vi "magnet ami connect.vi"(8 "error in (no error)":errorcluster, 10 "Z-Axis Communications Config":T1={"GPIB address"=22, "GPIB bus"=0, "connection ID"=refnum, "IP"="111.111.111.1", "Active Comm Interface"=0, "Serial Port"="", "Programmer Type"=0} {"Programmer Type" items=["Model 430", "Model 420"]; "Active Comm Interface" items=["TCP/IP (Model 430 Only)", "RS232", "IEEE488"]}, 11 "Y-Axis Communications Config":T1={"GPIB address"=22, "GPIB bus"=0, "connection ID"=refnum, "IP"="111.111.111.2", "Active Comm Interface"=0, "Serial Port"="", "Programmer Type"=0} {"Programmer Type" items=["Model 430", "Model 420"]; "Active Comm Interface" items=["TCP/IP (Model 430 Only)", "RS232", "IEEE488"]}) -> (0 "error out":errorcluster, 2 "Z-Axis Communications Config Out":T1={"GPIB address"=22, "GPIB bus"=0, "connection ID"=refnum, "IP"="111.111.111.1", "Active Comm Interface"=0, "Serial Port"="", "Programmer Type"=0} {"Programmer Type" items=["Model 430", "Model 420"]; "Active Comm Interface" items=["TCP/IP (Model 430 Only)", "RS232", "IEEE488"]}, 3 "Y-Axis Communications Config Out":T1={"GPIB address"=22, "GPIB bus"=0, "connection ID"=refnum, "IP"="111.111.111.2", "Active Comm Interface"=0, "Serial Port"="", "Programmer Type"=0} {"Programmer Type" items=["Model 430", "Model 420"]; "Active Comm Interface" items=["TCP/IP (Model 430 Only)", "RS232", "IEEE488"]})   [LabVIEW 2018]
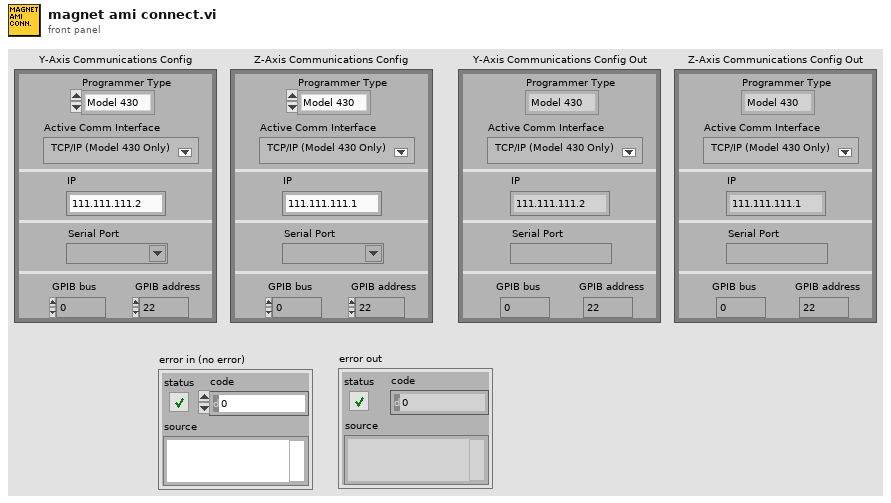
[diagram p1: front panel]
types:
  T1 = cluster{"GPIB address":i16, "GPIB bus":i16, "connection ID":refnum<k5>, "IP":string, "Active Comm Interface":u16, "Serial Port":refnum<visa-resource-name>, "Programmer Type":u16}
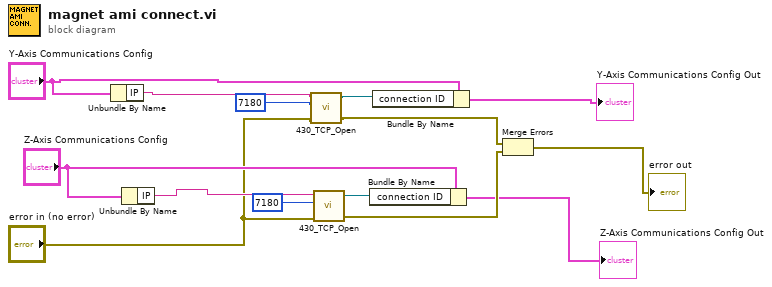
[diagram p0: block diagram]
diagram:
  n1 = Unbundle By Name("Y-Axis Communications Config") -> ("IP"=w8:string)
  n2 = Unbundle By Name("Z-Axis Communications Config") -> ("IP"=w6:string)
  n3 = call "430_TCP_Open.vi"("IP Address"=w8, "TCP Port"=7180, "error in (no error)"="error in (no error)") -> ("connection ID"=w10:refnum<k5>, "error out"=w9:errorcluster)  [unwired: 3 in, 1 out]
  n4 = call "430_TCP_Open.vi"("IP Address"=w6, "TCP Port"=7180, "error in (no error)"="error in (no error)") -> ("connection ID"=w13:refnum<k5>, "error out"=w12:errorcluster)  [unwired: 3 in, 1 out]
  n5 = Bundle By Name(cluster="Z-Axis Communications Config", "connection ID"=w13) -> (→"Z-Axis Communications Config Out":T1)
  n6 = Bundle By Name(cluster="Y-Axis Communications Config", "connection ID"=w10) -> (→"Y-Axis Communications Config Out":T1)
  n7 = Merge Errors(w9, w12) -> (→"error out":errorcluster)
